vi "Kalman_Filter_Initialize.vi"(8 "error in (no error)":errorcluster, 11 "Kalman_Filter in":refnum<class "Kalman_Filter.lvclass">) -> (0 "error out":errorcluster, 3 "Kalman_Filter out":refnum<class "Kalman_Filter.lvclass">)   [LabVIEW 2021, in "Kalman_Filter.lvclass"]
uses:
  Kalman_Filter.lvclass
  Kalman_Filter.lvclass/Kalman_Filter.ctl
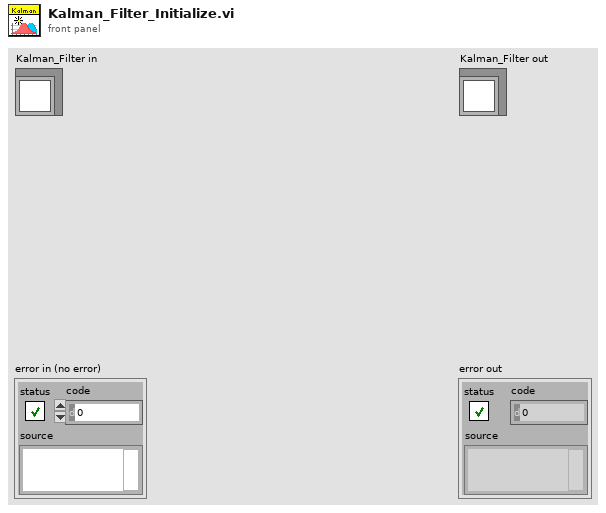
[diagram p1: front panel]
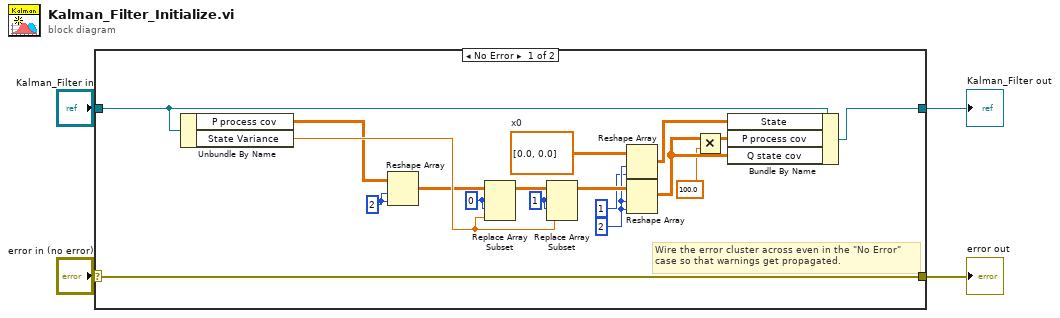
[diagram p0: block diagram]
diagram:
  n1 = case shown="No Error" "error in (no error)" {
    selector: "error in (no error)" -> [w22 w24]
    tunnel: [w22 w24] -> w3
    tunnel: [w16 w23] -> w1
    tunnel: "Kalman_Filter in" -> [w17 w23]
    frame No Error {
      w8 = 2 ("dimension size")
      w12 = 2
      w15 = 1 ("disabled index (col)")
      w13 = 0 ("index (row)")
      w21 = dbl[][] [[0.0], [0.0]]  # x0
      # "Wire the error cluster across even in the \"No Error\"\ncase so that warnings get propagated."
      n2 = Unbundle By Name(w17) -> ("P process cov"=w9:dbl[][], "State Variance"=w19:dbl)
      n3 = Reshape Array(w9, w8, w8) -> (w7:dbl[][])
      n4 = Replace Array Subset(array=w7, new element=w19, index (row)=w13, index (col)=w13) -> (w14:dbl[][])
      n5 = Replace Array Subset(array=w14, new element=w19, index (row)=w15, index (col)=w15) -> (w20:dbl[][])
      n6 = Reshape Array(w21, w12, 1) -> (w18:dbl[][])
      n7 = Reshape Array(w20, w12, w12) -> (w10:dbl[][])
      n8 = Multiply(x=w10, y=100.0) -> (x*y=w6:dbl[][])
      n9 = Bundle By Name(cluster=w17, "State"=w18, "P process cov"=w6, "Q state cov"=w10) -> (w16:refnum<class "Kalman_Filter.lvclass">)
    }
    frame Error {
    }
  }
  "error out" <- w3
  "Kalman_Filter out" <- w1
